vi "SeCrTs-Dequeue Message_R.vi"(8 "error in (no error)":errorcluster, 11 "Message Queue":refnum<queue>) -> (0 "error out":errorcluster, 1 "Message Data":variant, 2 "Message":string, 3 "dup Message Queue":refnum<queue>)   [LabVIEW 2022 SP3]
uses:
  RT Controls/SeCrTs-Message Cluster_R.ctl
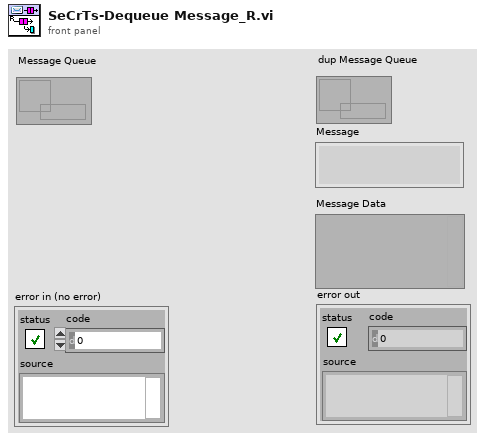
[diagram p1: front panel]
types:
  T1 = typedef "SeCrTs-Message Cluster_R.ctl" = cluster{"Message":string, "Message Data":variant}
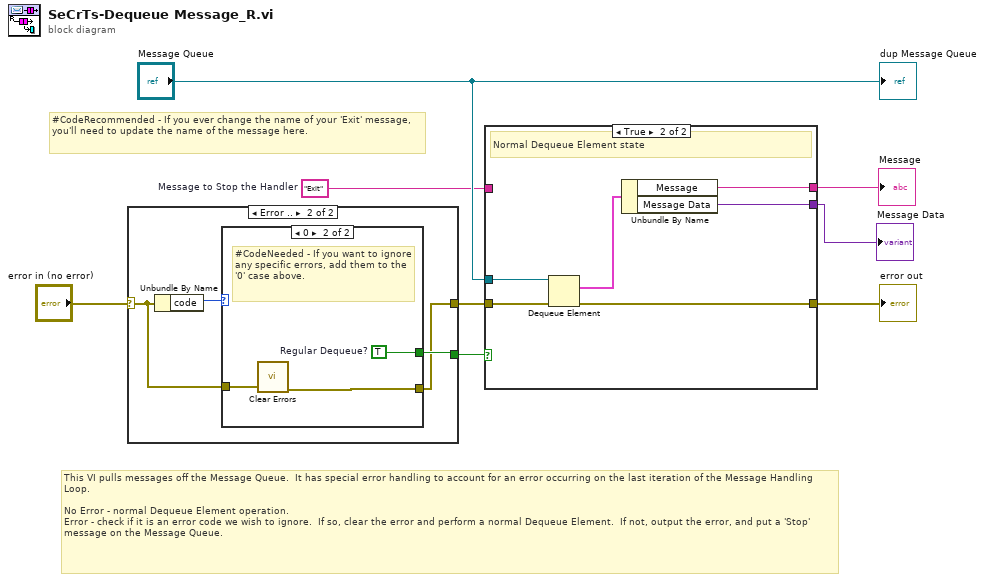
[diagram p0: block diagram]
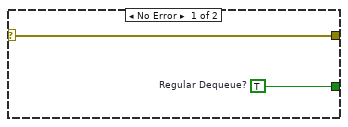
[diagram p2: hidden frame]
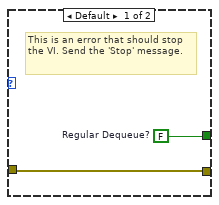
[diagram p3: hidden frame]
diagram:
  w1 = "Exit"  # Message to Stop the Handler
  # "#CodeRecommended - If you ever change the name of your 'Exit' message, you'll need to update the name of the message here."
  # "This VI pulls messages off the Message Queue.  It has special error handling to account for an error occurring on the last iteration of the Message Handling Loop.\n\nNo Error - normal Dequeue Element operation.\nError - check if it is an error code we wish to ignore.  If so, clear the error and perform a normal Dequeue Element.  If not, output the error, and put a 'Stop' message on the Message Queue."
  n1 = case shown="Error .." "error in (no error)" {
    selector: "error in (no error)" -> [w10 w13]
    tunnel: [w10 w12] -> w5
    tunnel: [w9 w14] -> w4
    frame No Error {
      w9 = TRUE  # Regular Dequeue?
    }
    frame Error {
      n2 = Unbundle By Name(w13) -> ("code"=w11:i32)
      n3 = case shown="0" w11 {
        tunnel: [w15 w19] -> w14
        tunnel: w13 -> [w16 w18]
        tunnel: [w16 w17] -> w12
        frame Default {
          w15 = FALSE  # Regular Dequeue?
          # "This is an error that should stop the VI. Send the 'Stop' message."
        }
        frame 0 {
          w19 = TRUE  # Regular Dequeue?
          # "#CodeNeeded - If you want to ignore any specific errors, add them to the '0' case above."
          n4 = call <vilib>:"Clear Errors.vi"("error in (no error)"=w18) -> ("error out"=w17:errorcluster)  [unwired: 5 in, 1 out]
        }
      }
    }
  }
  n5 = case shown="True" w4 {
    tunnel: [w20 w27] -> w8
    tunnel: "Message Queue" -> [_ w26]
    tunnel: w5 -> [w20 w25]
    tunnel: [w21 w23] -> w3
    tunnel: [_ w22] -> w2
    tunnel: w1 -> [w21 _]
    frame False {
      # "Error"
    }
    frame True {
      # "Normal Dequeue Element state"
      n6 = Dequeue Element(queue=w26, error in (no error)=w25) -> (element=w24:T1, error out=w27:errorcluster)  [unwired: 1 in, 2 out]
      n7 = Unbundle By Name(w24) -> ("Message"=w23:string, "Message Data"=w22:variant)
    }
  }
  "error out" <- w8
  "Message" <- w3
  "Message Data" <- w2
  "dup Message Queue" <- "Message Queue"
